vi "Save Spectral Data.vi"(7 "#A lines":i32=1250, 9 "file path":path, 10 "#B lines":i32, 11 "data in":u16[][](array[numeric])) -> ()   [LabVIEW 2018]
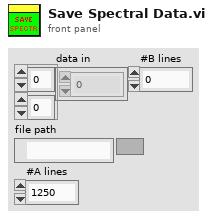
[diagram p1: front panel]
types:
  T1 = enum16{"big-endian, network order", "native, host order", "little-endian"}
  T2 = enum16{"open", "replace", "create", "open or create", "replace or create", "replace or create with confirmation"}
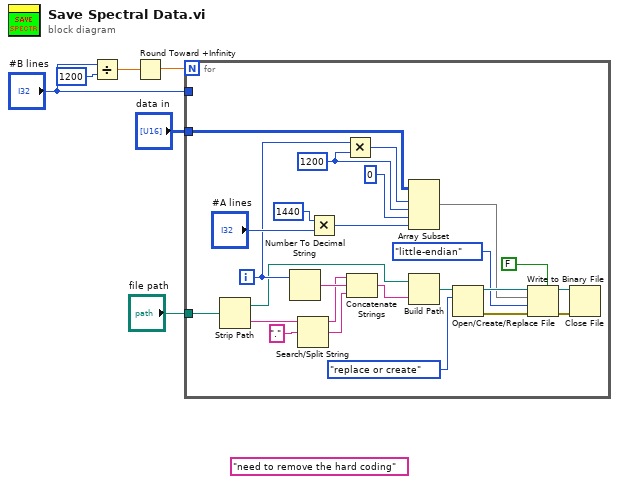
[diagram p0: block diagram]
diagram:
  (unwired) "need to remove the hard coding"
  n1 = Divide(x="#B lines", y=1200) -> (x/y=w5:dbl)
  n2 = Round Toward +Infinity(x=w5) -> (ceil(x): smallest int >= x=w4:dbl)
  n3 = for {
    N: w4 -> [_]
    tunnel: "file path" -> [w12]
    tunnel: "data in" -> [w25]
    tunnel: "#B lines" -> [_]
    i -> [w15]
    w13 = 1200 ("y")
    n4 = Strip Path(path=w12) -> (stripped path=w11:path, name=w10:string)
    n5 = Number To Decimal String(number=w15) -> (decimal integer string=w17:string)  [unwired: 1 in]
    n6 = Search/Split String(string=w10, search string/char (-)=".") -> (substring before match=w8:string, match + rest of string=w7:string)  [unwired: 1 in, 1 out]
    n7 = Multiply(x=1440, y="#A lines") -> (x*y=w18:i32)
    n8 = Multiply(x=w15, y=w13) -> (x*y=w14:i32)
    n9 = Concatenate Strings(w8, w17, w7) -> (w16:string)
    n10 = Array Subset(array=w25, index (row)=w14, length (row)=w13, index (col)=0 ("index"), length (col)=w18) -> (w23:u16[][])
    n11 = Build Path(base path=w11, name or relative path=w16) -> (appended path=w21:path)
    n12 = Open/Create/Replace File(file path (use dialog)=w21, operation (0:open)=T2."replace or create") -> (refnum out=w27:refnum<file>, error out=w29:errorcluster)  [unwired: 4 in, 1 out]
    n13 = Write to Binary File(file (use dialog)=w27, data=w23, error in=w29, 5:FALSE ("prepend array or string size? (T)"), 9:T1."little-endian" ("byte order (0:big-endian, network order)")) -> (refnum out=w26:refnum<file>, error out=w28:errorcluster)  [unwired: 1 in, 1 out]
    n14 = Close File(refnum=w26, error in=w28) -> ()  [unwired: 2 out]
  }
